vi "test aceleration CMP sensor - injection.vi"() -> ()   [LabVIEW 2013]
uses:
  <vilib>/measure/maspectr.llb/Power Spectrum and PSD Export Mode.ctl
  <vilib>/DAQmx/read.llb/DAQmx Read (Analog 1D Wfm NChan NSamp).vi
  <vilib>/Analysis/2dsp.llb/Real FFT.vi
  <vilib>/Analysis/2dsp.llb/Power Spectrum (DBL).vi
  <vilib>/DAQmx/create/channels.llb/DAQmx Create Channel (AI-Voltage-Basic).vi
  <vilib>/DAQmx/configure/timing.llb/DAQmx Timing (Sample Clock).vi
  <vilib>/measure/mamon.llb/Trigger Detection for 1 Channel.vi
  <vilib>/Waveform/WDTOps.llb/WDT Get Waveform Subset DBL.vi
  <vilib>/measure/mascope.llb/Pulse Measurements 1 chan.vi
  <vilib>/DAQmx/miscellaneous.llb/DAQmx Fill In Error Info.vi
  <vilib>/measure/maspectr.llb/FFT Power Spectrum and PSD for 1 Chan.vi
  <vilib>/measure/maspectr.llb/FFT Spectrum (Mag-Phase) for 1 Chan.vi
  <vilib>/measure/maspectr.llb/FFT Spectrum (Real-Im) for 1 Chan.vi
  <vilib>/measure/NI_MAPro.lvlib
  <resource>/objmgr/daqmx.rc
  <vilib>/Analysis/NI_AALPro.lvlib
panel:
  out "error out 2":errorcluster
  out "element":string
  in  "index (row)":i32
  in  "spectrum units table":string[][](table)=[["FFT", "N * V", "N/2 * Vpk"], ["Power Spectrum", "V^2", "1/2 * Vrms^2"], ["Auto Power Spectrum", "V^2", "Vrms^2"], ["Amplitude and Phase Spectrum", "V", "Vrms"], ["FFT Power Spectrum", "V^2", "Vrms^2"], ["FFT Power Spectral Density", "V^2/Hz", "Vrms^2/Hz"], ["FFT Spectrum (Mag-Phase)", "V", "Vrms"], ["FFT Spectrum (Real-Imag)", "V", "Vrms"]]
  in  "stop 2":bool
  out "spectral plot":cluster{"t":dbl, "t":dbl, "magnitude":dbl[]}(graph)={"t"=0.0, "t"=1.0, "magnitude"=[]}
  out "Waveform Graph 2":dynamicdata(graph)
  out "trigger location":dbl format="%#_2g"
  out "fs":dbl
  out "rpm":dbl
  out "period":dbl format="%.2g"
  out "error out":errorcluster
  out "f":dbl
  out "Waveform Graph 3":waveform(dbl)(graph)
  out "Waveform Graph":waveform(dbl)[](graph)
  in  "stop":bool
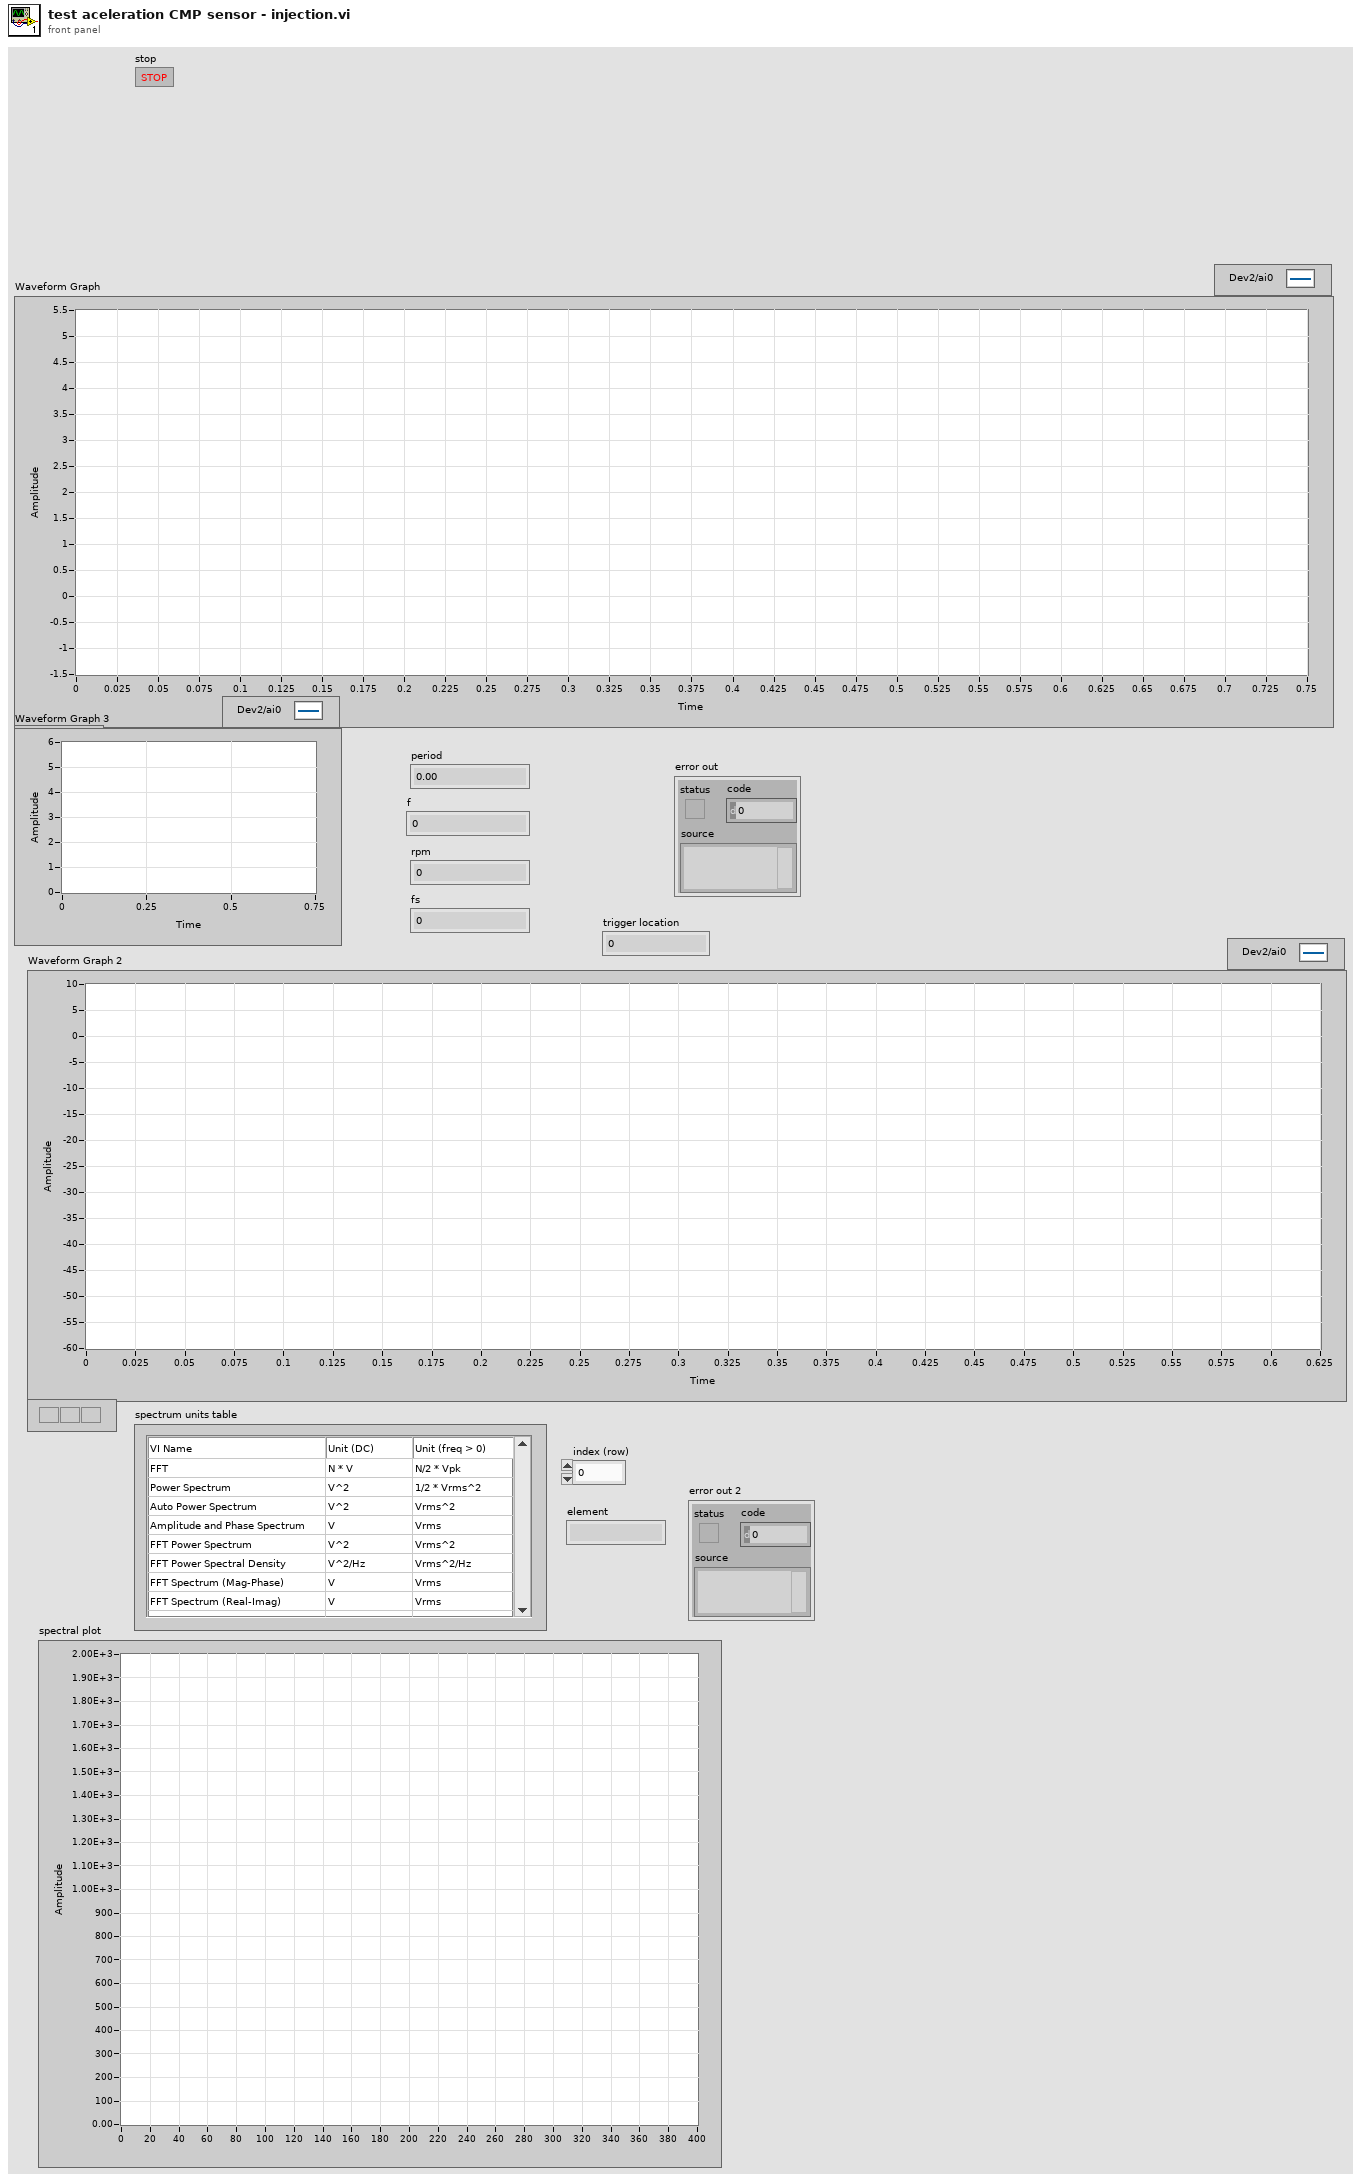
[diagram p1: front panel]
types:
  T1 = enum16{"None ", "Hanning", "Hamming", "Blackman-Harris", "Exact Blackman", "Blackman", "Flat Top", "4 Term B-Harris ", "7 Term B-Harris", "Low Sidelobe"}
  T2 = cluster{"dB On (F)":bool, "unwrap phase (F)":bool, "convert to degree (F)":bool}
  T3 = typedef "NI_MAPro.lvlib/Power Spectrum and PSD Export Mode.ctl" = u16
  T4 = cluster{"f0":dbl, "df":dbl, "imaginary part":dbl[]}
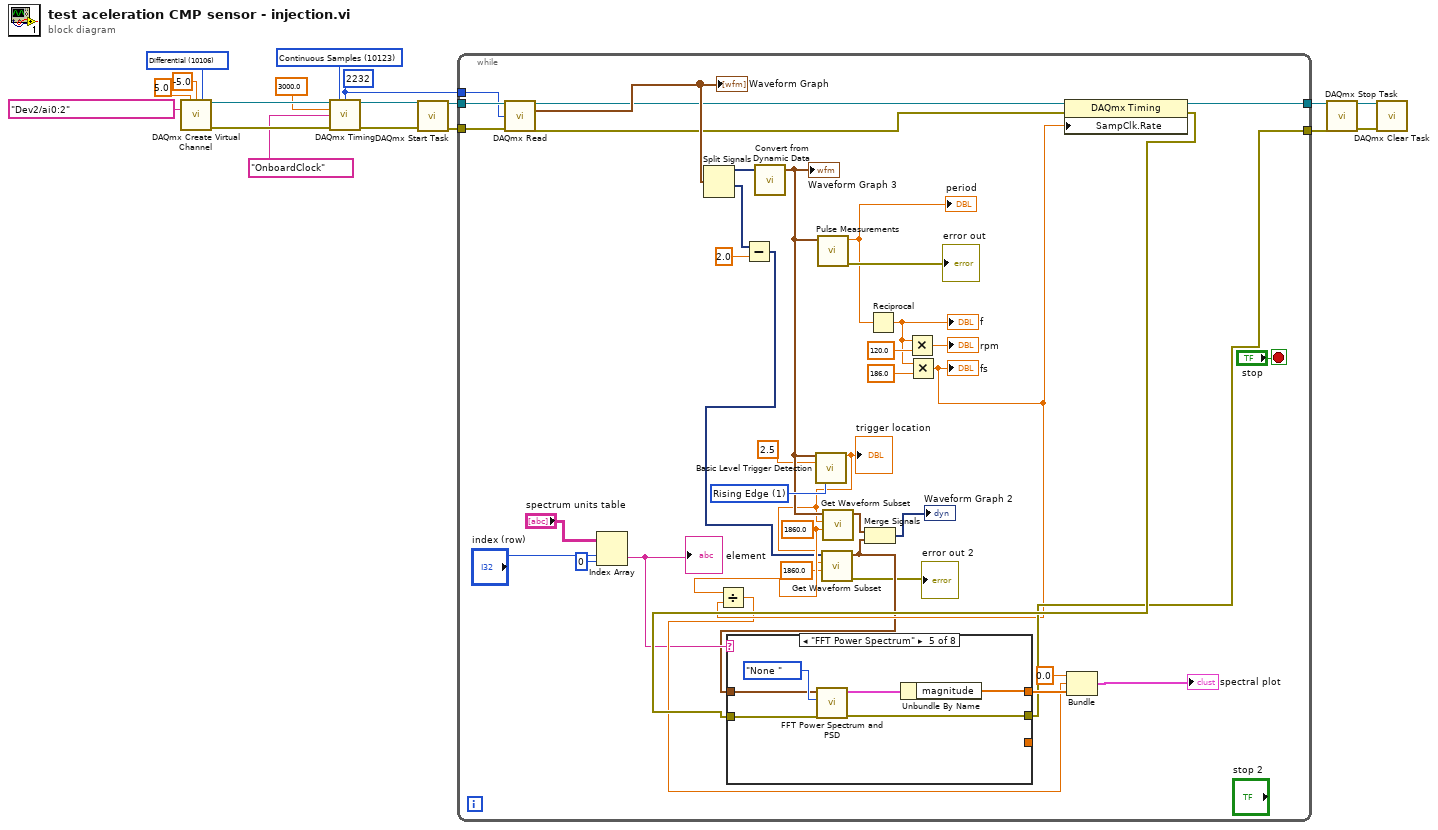
[diagram p0: block diagram]
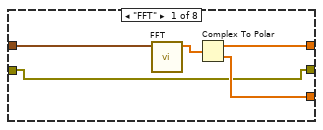
[diagram p2: hidden frame]
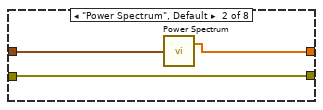
[diagram p3: hidden frame]
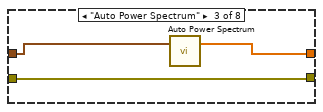
[diagram p4: hidden frame]
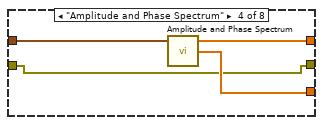
[diagram p5: hidden frame]
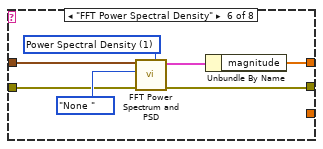
[diagram p6: hidden frame]
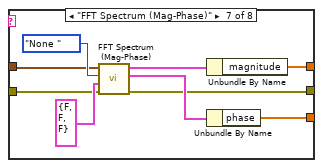
[diagram p7: hidden frame]
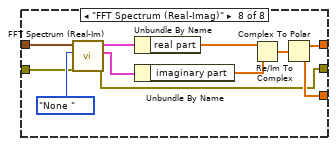
[diagram p8: hidden frame]
diagram:
  w7 = 10123 items=["Finite Samples"=10178, "Continuous Samples"=10123, "Hardware Timed Single Point"=12522] ("sample mode")
  w5 = 2232 ("samples per channel")
  w15 = 10106 items=["default"=-1, "RSE"=10083, "NRSE"=10078, "Differential"=10106, "Pseudodifferential"=12529] ("input terminal configuration")
  n1 = call-poly <vilib>:"DAQmx Create Virtual Channel.vi"("maximum value"=5.0, "minimum value"=-5.0, "input terminal configuration"=w15, "physical channels"=tag "Dev2/ai0:2") -> ("task out"=w14:refnum<k21>, "error out"=w13:errorcluster)  [unwired: 5 in, 5 out]
  n2 = call-poly <vilib>:"DAQmx Timing.vi"("task/channels in"=w14, "sample mode"=w7, "samples per channel"=w5, "rate"=3000.0, "source"=tag "OnboardClock", "error in"=w13) -> ("task out"=w12:refnum<k21>, "error out"=w11:errorcluster)  [unwired: 1 in, 7 out]
  n3 = call <vilib>:"DAQmx Start Task.vi"("task/channels in"=w12, "error in"=w11) -> ("task out"=w10:refnum<k21>, "error out"=w8:errorcluster)  [unwired: 12 out]
  n4 = while {
    tunnel: w8 -> [w57]
    tunnel: w10 -> [w56]
    tunnel: [w47] -> w4
    tunnel: [w40] -> w1
    tunnel: w5 -> [w25]
    stop <- "stop" stop-if-true
    w39 = 1860.0 ("duration")
    w46 = u16 1 items=["Falling Edge", "Rising Edge"] ("trigger slope")
    n5 = call-poly <vilib>:"DAQmx Read.vi"("task/channels in"=w56, "number of samples per channel"=w25, "error in"=w57) -> ("task out"=w23:refnum<k21>, "data"=w54:waveform(dbl)[], "error out"=w24:errorcluster)  [unwired: 10 out]
    "Waveform Graph" <- w54
    n6 = Index Array(array="spectrum units table", index (row)="index (row)", index (col)=0 ("disabled index (col)")) -> (element=w33:string)
    "element" <- w33
    n7 = Split Signals(w54) -> (w22:dynamicdata, w21:dynamicdata)  [unwired: 4 in, 2 out]
    n8 = Subtract(x=w21, y=2.0) -> (x-y=w19:dynamicdata)
    n9 = call "Convert from Dynamic Data"("Dynamic Data Type"=w22) -> ("Waveform"=w45:waveform(dbl))  [unwired: 3 in]
    "Waveform Graph 3" <- w45
    n10 = call-poly <vilib>:"Basic Level Trigger Detection.vi"("signal in"=w45, "level"=2.5, "trigger slope"=w46) -> ("trigger location"=w31:dbl)  [unwired: 10 in, 2 out]
    "trigger location" <- w31
    n11 = call-poly <vilib>:"Pulse Measurements.vi"("signal in"=w45) -> ("error out"=→"error out":errorcluster, "period"=w49:dbl)  [unwired: 6 in, 3 out]
    "period" <- w49
    n12 = call-poly <vilib>:"Get Waveform Subset.vi"("duration"=1860.0, "start samples/time"=w31, "waveform in"=w19) -> ("error out"=→"error out 2":errorcluster, "waveform out"=w29:waveform(dbl))  [unwired: 3 in, 2 out]
    n13 = call-poly <vilib>:"Get Waveform Subset.vi"("duration"=w39, "start samples/time"=w31, "waveform in"=w45) -> ("waveform out"=w30:waveform(dbl))  [unwired: 3 in, 3 out]
    n14 = Merge Signals(w30, w29) -> (→"Waveform Graph 2":dynamicdata)
    n15 = Reciprocal(x=w49) -> (1/x=w48:dbl)
    "f" <- w48
    n16 = Multiply(x=w48, y=120.0) -> (x*y=→"rpm":dbl)
    n17 = Multiply(x=w48, y=186.0) -> (x*y=w38:dbl)
    "fs" <- w38
    n18 = Divide(x=w39, y=w38) -> (x/y=w37:dbl)
    n19 = property class="DAQmx Timing"(reference=w23, error in=w24, "SampClk.Rate"=w38) -> (reference out=w47:refnum<k21>, error out=w41:errorcluster)
    n20 = case shown="\"FFT Power Spectrum\"" w33 {
      tunnel: [w61 w65 w68 w72 w77 w84 w93 w99] -> w43
      tunnel: [w60 _ _ w71 _ _ w90 w98] -> _
      tunnel: [w58 w63 w66 w69 w75 w81 w88 w97] -> w40
      tunnel: w29 -> [w59 w64 w67 w70 w74 w80 w86 w96]
      tunnel: w41 -> [w58 w63 w66 w69 w73 w79 w87 w95]
      frame "FFT" {
        n21 = call-poly <vilib>:"FFT.vi"("X"=w59) -> ("FFT {X}"=w62:cdb[])  [unwired: 9 in, 1 out]
        n22 = Complex To Polar(r * e^(i*theta)=w62) -> (r=w61:dbl[], theta=w60:dbl[])
      }
      frame "Power Spectrum", Default {
        n23 = call-poly <vilib>:"Power Spectrum.vi"("X"=w64) -> ("Power Spectrum"=w65:dbl[])  [unwired: 1 out]
      }
      frame "Auto Power Spectrum" {
        n24 = call <vilib>:"Auto Power Spectrum.vi"("Signal (V)"=w67) -> ("Power Spectrum (V^2 rms)"=w68:dbl[])  [unwired: 1 in, 1 out]
      }
      frame "Amplitude and Phase Spectrum" {
        n25 = call <vilib>:"Amplitude and Phase Spectrum.vi"("Signal (V)"=w70) -> ("Amp Spectrum Phase (radians)"=w71:dbl[], "Amp Spectrum Mag (Vrms)"=w72:dbl[])  [unwired: 2 in, 1 out]
      }
      frame "FFT Power Spectrum" {
        n26 = call-poly <vilib>:"FFT Power Spectrum and PSD.vi"("error in (no error)"=w73, "window"=T1."None ", "time signal"=w74) -> ("error out"=w75:errorcluster, "Power Spectrum / PSD"=w78:cluster{"f0":dbl, "df":dbl, "magnitude":dbl[]})  [unwired: 5 in, 2 out]
        n27 = Unbundle By Name(w78) -> ("magnitude"=w77:dbl[])
      }
      frame "FFT Power Spectral Density" {
        w82 = T3 1 items=["Power Spectrum", "Power Spectral Density"] ("export mode")
        n28 = call-poly <vilib>:"FFT Power Spectrum and PSD.vi"("export mode"=w82, "error in (no error)"=w79, "window"=T1."None ", "time signal"=w80) -> ("error out"=w81:errorcluster, "Power Spectrum / PSD"=w85:cluster{"f0":dbl, "df":dbl, "magnitude":dbl[]})  [unwired: 4 in, 2 out]
        n29 = Unbundle By Name(w85) -> ("magnitude"=w84:dbl[])
      }
      frame "FFT Spectrum (Mag-Phase)" {
        n30 = call-poly <vilib>:"FFT Spectrum (Mag-Phase).vi"("error in (no error)"=w87, "view"=T2 {"dB On (F)"=FALSE, "unwrap phase (F)"=FALSE, "convert to degree (F)"=FALSE}, "window"=T1."None ", "time signal"=w86) -> ("error out"=w88:errorcluster, "phase"=w91:cluster{"f0":dbl, "df":dbl, "phase":dbl[]}, "magnitude"=w94:cluster{"f0":dbl, "df":dbl, "magnitude":dbl[]})  [unwired: 3 in, 2 out]
        n31 = Unbundle By Name(w94) -> ("magnitude"=w93:dbl[])
        n32 = Unbundle By Name(w91) -> ("phase"=w90:dbl[])
      }
      frame "FFT Spectrum (Real-Imag)" {
        n33 = call-poly <vilib>:"FFT Spectrum (Real-Im).vi"("error in (no error)"=w95, "window"=T1."None ", "time signal"=w96) -> ("error out"=w97:errorcluster, "imaginary part"=w103:T4, "real part"=w105:cluster{"f0":dbl, "df":dbl, "real part":dbl[]})  [unwired: 4 in, 2 out]
        n34 = Unbundle By Name(w105) -> ("real part"=w102:dbl[])
        n35 = Unbundle By Name(w103) -> ("imaginary part"=w101:dbl[])
        n36 = Re/Im To Complex(1:w101, 2:w102) -> (0:w100:cdb[])
        n37 = Complex To Polar(r * e^(i*theta)=w100) -> (r=w99:dbl[], theta=w98:dbl[])
      }
    }
    n38 = Bundle("t"=0.0, w37, "magnitude"=w43) -> (→"spectral plot":cluster{"t":dbl, dbl, "magnitude":dbl[]})  [unwired: 1 in]
  }
  n39 = call <vilib>:"DAQmx Stop Task.vi"("task/channels in"=w4, "error in"=w1) -> ("task out"=w3:refnum<k21>, "error out"=w2:errorcluster)  [unwired: 12 out]
  n40 = call <vilib>:"DAQmx Clear Task.vi"("task in"=w3, "error in"=w2) -> ()  [unwired: 13 in, 1 out]
